vi "Generic command handler.vi"(8 "error in (no error)":errorcluster, 10 "Message in":refnum<class "GenericMessage.lvclass">, 11 "Retiga in":refnum<class "Retiga.lvclass">) -> (0 "error out":errorcluster, 2 "value":string, 3 "Retiga out":refnum<class "Retiga.lvclass">)   [LabVIEW 2012, in "Retiga.lvclass"]
doc: "The generic_command_handler processes the command 'generic'. Commands which are not part of the predefined list of commands fall under the 'generic' command for special activity."
uses:
  Retiga.lvclass
  <vilib>/Distrio/Murmex/GenericMessage/GenericMessage.lvclass
  <vilib>/Distrio/Murmex/Murmex/Murmex.lvclass
  Retiga.lvclass/Retiga.ctl
  <vilib>/Distrio/Murmex/ProceedMessage/ProceedMessage.lvclass
panel:
  # "This method is called when the GENERIC\ntrigger is sent. \n\nOverride this method when your component needs to\nrespond to this trigger. \n\nCall parent for proper implementation"
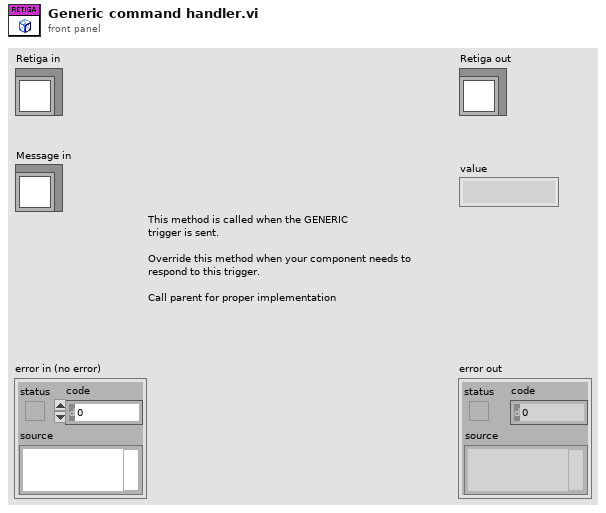
[diagram p1: front panel]
types:
  T1 = typedef "IMAQ Image.ctl" = refnum<image>
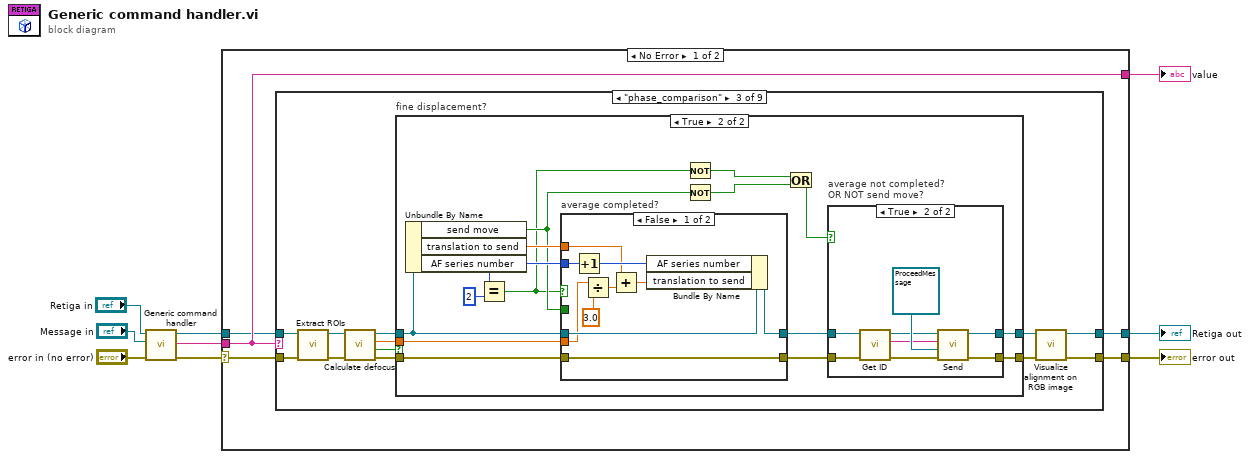
[diagram p0: block diagram]
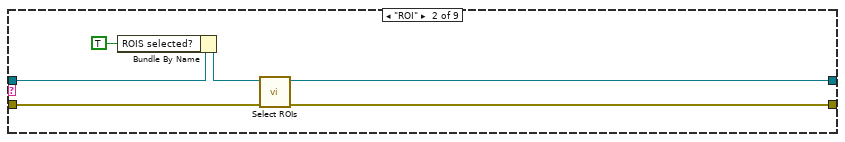
[diagram p3: hidden frame]
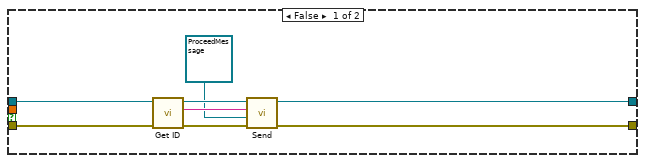
[diagram p4: hidden frame]
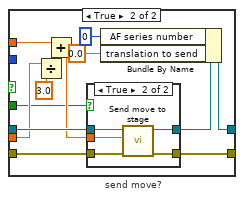
[diagram p6: hidden frame]
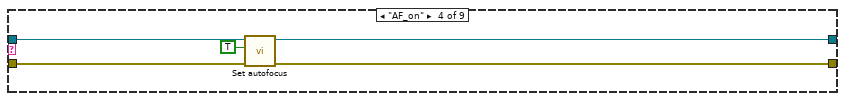
[diagram p8: hidden frame]
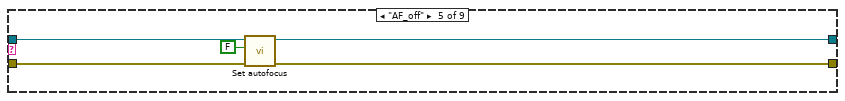
[diagram p9: hidden frame]
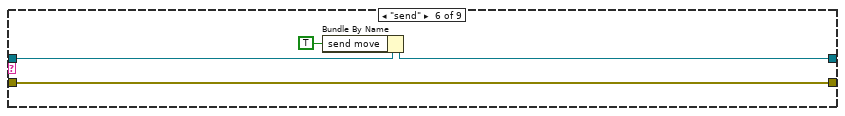
[diagram p10: hidden frame]
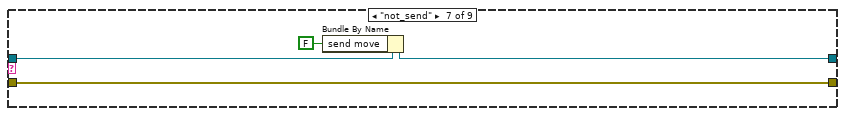
[diagram p11: hidden frame]
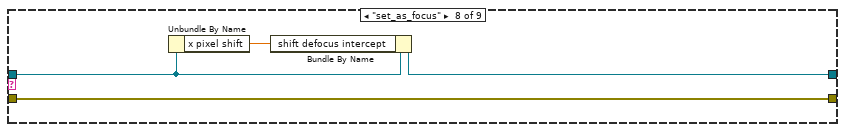
[diagram p12: hidden frame]
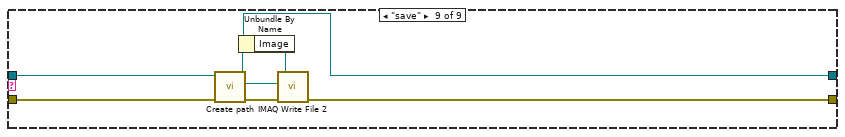
[diagram p13: hidden frame]
diagram:
  n1 = call-parent "Generic command handler.vi"("error in (no error)"="error in (no error)", "Message in"="Message in", "Murmex in"="Retiga in") -> ("error out"=w6:errorcluster, "value"=w4:string, "Murmex out"=w5:refnum<class "Retiga.lvclass">)  [unwired: 6 in]
  n2 = case shown="No Error" w6 {
    selector: w6 -> [w12 w128]
    tunnel: w5 -> [w10 w129]
    tunnel: w4 -> [w14 w127]
    tunnel: [w11 w129] -> w3
    tunnel: [w13 w128] -> w2
    tunnel: [w14 w127] -> w1
    frame No Error {
      n3 = case shown="\"phase_comparison\"" w14 {
        tunnel: [w16 w18 w26 w99 w104 w109 w113 w116 w121] -> w13
        tunnel: w12 -> [w16 w19 w33 w102 w107 w109 w113 w116 w125]
        tunnel: [w15 w17 w24 w100 w105 w110 w114 w117 w120] -> w11
        tunnel: w10 -> [w15 w22 w34 w101 w106 w111 w115 w119 w126]
        frame Default {
        }
        frame "ROI" {
          n4 = Bundle By Name(cluster=w22, "ROIS selected?"=TRUE ("runtime.ROIS selected?")) -> (w20:refnum<class "Retiga.lvclass">)
          n5 = call-dynamic "Select ROIs.vi"("error in (no error)"=w19, "Retiga in"=w20) -> ("error out"=w18:errorcluster, "Retiga out"=w17:refnum<class "Retiga.lvclass">)  [unwired: 8 in]
        }
        frame "phase_comparison" {
          n6 = call-dynamic "Extract ROIs.vi"("error in (no error)"=w33, "Retiga in"=w34) -> ("error out"=w31:errorcluster, "Retiga out"=w32:refnum<class "Retiga.lvclass">)  [unwired: 8 in]
          n7 = call-dynamic "Calculate defocus.vi"("error in (no error)"=w31, "Retiga in"=w32) -> ("error out"=w29:errorcluster, "fine?"=w23:bool, "translation out"=w30:dbl[unit], "Retiga out"=w28:refnum<class "Retiga.lvclass">)  [unwired: 6 in]
          n8 = case "fine displacement?" shown="True" w23 {
            tunnel: w30 -> [_ w53]
            tunnel: w29 -> [w40 w57]
            tunnel: w28 -> [w38 w56]
            tunnel: [w41 w50] -> w25
            tunnel: [w42 w48] -> w27
            frame False {
              n9 = call <vilib>:"Get ID.vi"("error in (no error)"=w40, "Murmex in"=w38) -> ("error out"=w39:errorcluster, "component id"=w36:string, "Murmex out"=w37:refnum<class "Retiga.lvclass">)  [unwired: 7 in]
              n10 = call <vilib>:"Send.vi"("error in (no error)"=w39, "Message"=refnum<class "ProceedMessage.lvclass"> refnum ("Distrio Murmex 1.5:ProceedMessage"), "recipient"=w36, "Murmex in"=w37) -> ("error out"=w42:errorcluster, "Murmex out"=w41:refnum<class "Retiga.lvclass">)  [unwired: 6 in]
            }
            frame True {
              n11 = Unbundle By Name(w56) -> ("send move"=w51:bool, "translation to send"=w52:dbl[unit], "AF series number"=w54:i32)
              n12 = Equal?(x=w54, y=2) -> (x = y?=w46:bool)
              n13 = case "average completed?" shown="False" w46 {
                tunnel: w56 -> [w75 w90]
                tunnel: [w76 w81] -> w49
                tunnel: w57 -> [w73 w89]
                tunnel: [w73 w88] -> w47
                tunnel: w54 -> [w77 _]
                tunnel: w53 -> [w68 w84]
                tunnel: w52 -> [w71 w85]
                tunnel: w51 -> [_ w78]
                frame False {
                  n14 = Increment(x=w77) -> (x+1=w74:i32)
                  n15 = Divide(x=w68, y=3.0) -> (x/y=w70:dbl[unit])
                  n16 = Add(x=w71, y=w70) -> (x+y=w69:dbl[unit])
                  n17 = Bundle By Name(cluster=w75, "AF series number"=w74, "translation to send"=w69) -> (w76:refnum<class "Retiga.lvclass">)
                }
                frame True {
                  n18 = Divide(x=w84, y=3.0) -> (x/y=w87:dbl[unit])
                  n19 = Add(x=w85, y=w87) -> (x+y=w83:dbl[unit])
                  n20 = case "send move?" shown="True" w78 {
                    tunnel: w90 -> [w92 w97]
                    tunnel: w89 -> [w91 w96]
                    tunnel: [w91 w95] -> w88
                    tunnel: w83 -> [_ w94]
                    tunnel: [w92 w93] -> w82
                    frame False {
                    }
                    frame True {
                      n21 = call-dynamic "Send move to stage.vi"("error in (no error)"=w96, "move to send"=w94, "Retiga in"=w97) -> ("error out"=w95:errorcluster, "Retiga out"=w93:refnum<class "Retiga.lvclass">)  [unwired: 7 in]
                    }
                  }
                  n22 = Bundle By Name(cluster=w82, "AF series number"=0 ("runtime.AF series number"), "translation to send"=dbl[unit] 0.0 ("runtime.translation to send")) -> (w81:refnum<class "Retiga.lvclass">)
                }
              }
              n23 = Not(x=w46) -> (.not. x?=w45:bool)
              n24 = Not(x=w51) -> (.not. x?=w44:bool)
              n25 = Or(x=w45, y=w44) -> (x .or. y?=w43:bool)
              n26 = case "average not completed? \nOR NOT send move?" shown="True" w43 {
                tunnel: [w59 w61] -> w50
                tunnel: w49 -> [w59 w63]
                tunnel: [w58 w60] -> w48
                tunnel: w47 -> [w58 w62]
                frame False {
                }
                frame True {
                  n27 = call <vilib>:"Get ID.vi"("error in (no error)"=w62, "Murmex in"=w63) -> ("error out"=w64:errorcluster, "component id"=w66:string, "Murmex out"=w65:refnum<class "Retiga.lvclass">)  [unwired: 7 in]
                  n28 = call <vilib>:"Send.vi"("error in (no error)"=w64, "Message"=refnum<class "ProceedMessage.lvclass"> refnum ("Distrio Murmex 1.5:ProceedMessage"), "recipient"=w66, "Murmex in"=w65) -> ("error out"=w60:errorcluster, "Murmex out"=w61:refnum<class "Retiga.lvclass">)  [unwired: 6 in]
                }
              }
            }
          }
          n29 = call-dynamic "Visualize alignment on RGB image.vi"("error in (no error)"=w27, "Retiga in"=w25) -> ("error out"=w26:errorcluster, "Retiga out"=w24:refnum<class "Retiga.lvclass">)  [unwired: 8 in]
        }
        frame "AF_on" {
          n30 = call-dynamic "Set autofocus.vi"("error in (no error)"=w102, "autofocusing?"=TRUE, "Retiga in"=w101) -> ("error out"=w99:errorcluster, "Retiga out"=w100:refnum<class "Retiga.lvclass">)  [unwired: 7 in]
        }
        frame "AF_off" {
          n31 = call-dynamic "Set autofocus.vi"("error in (no error)"=w107, "autofocusing?"=FALSE, "Retiga in"=w106) -> ("error out"=w104:errorcluster, "Retiga out"=w105:refnum<class "Retiga.lvclass">)  [unwired: 7 in]
        }
        frame "send" {
          n32 = Bundle By Name(cluster=w111, "send move"=TRUE ("runtime.cross correlation.send move")) -> (w110:refnum<class "Retiga.lvclass">)
        }
        frame "not_send" {
          n33 = Bundle By Name(cluster=w115, "send move"=FALSE ("runtime.cross correlation.send move")) -> (w114:refnum<class "Retiga.lvclass">)
        }
        frame "set_as_focus" {
          n34 = Unbundle By Name(w119) -> ("x pixel shift"=w118:dbl)
          n35 = Bundle By Name(cluster=w119, "shift defocus intercept"=w118) -> (w117:refnum<class "Retiga.lvclass">)
        }
        frame "save" {
          n36 = call-dynamic "Create path.vi"("error in (no error)"=w125, "Retiga in"=w126) -> ("error out"=w122:errorcluster, "full path"=w123:path, "Retiga out"=w120:refnum<class "Retiga.lvclass">)  [unwired: 7 in]
          n37 = Unbundle By Name(w120) -> ("Image"=w124:T1)
          n38 = call-poly "IMAQ Write File 2"("error in (no error)"=w122, "File Path"=w123, "Image"=w124) -> ("error out"=w121:errorcluster)  [unwired: 7 in, 1 out]
        }
      }
    }
    frame Error {
    }
  }
  "error out" <- w2
  "Retiga out" <- w3
  "value" <- w1
